vi "delete_element.vi"(10 "element":i32, 11 "array in":i32[](array[numeric])) -> (3 "array out":i32[](array[numeric]))   [LabVIEW 2015, in "PolyVIEW.lvclass"]
uses:
  PolyVIEW.lvclass
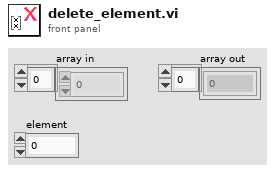
[diagram p1: front panel]
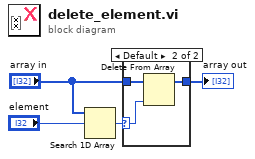
[diagram p0: block diagram]
diagram:
  n1 = Search 1D Array(1D array="array in", element="element") -> (index of element=w1:i32)  [unwired: 1 in]
  n2 = case shown="Default" w1 {
    selector: w1 -> [_ w7]
    tunnel: "array in" -> [w5 w8]
    tunnel: [w5 w6] -> w4
    frame -1 {
    }
    frame Default {
      n3 = Delete From Array(array=w8, index=w7) -> (array with subset deleted=w6:i32[])  [unwired: 1 in, 1 out]
    }
  }
  "array out" <- w4
